vi "Test_WriteCluster_CheckDisk_ValuePresent.vi"(8 "error in (no error)":errorcluster, 11 "TestCase in":refnum<class "TestPersistToDiskTransport.lvclass">) -> (0 "error out":errorcluster, 3 "TestCase out":refnum<class "TestPersistToDiskTransport.lvclass">)   [LabVIEW 2017, in "TestPersistToDiskTransport.lvclass"]
uses:
  TestPersistToDiskTransport.lvclass
  TestPersistToDiskTransport.lvclass/TestPersistToDiskTransport.ctl
  Source/Concrete/PersistToDiskTransport/PersistToDiskTransport.lvclass/PersistToDiskTransport.ctl
  <vilib>/Utility/error.llb/Clear Errors.vi
  Source/Concrete/PersistToDiskTransport/Format Persistent Filename.vi
  Source/Concrete/PersistToDiskTransport/PersistToDiskTransport.lvclass
  C:/Git/composed-transport/Source/ITransport/ITransport.lvclass
  externals/variant-extensions/Source/Format Type String.vi
  Source/ITransport/ITransport.lvclass
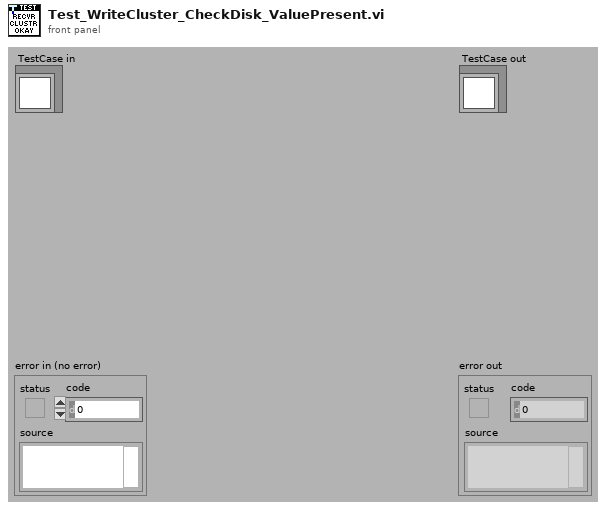
[diagram p1: front panel]
types:
  T1 = typedef "PersistToDiskTransport.lvclass/Recovered Value.ctl" = cluster{"Datum Name":string, "Datum Value":variant, "Last Publication Time":timestamp}
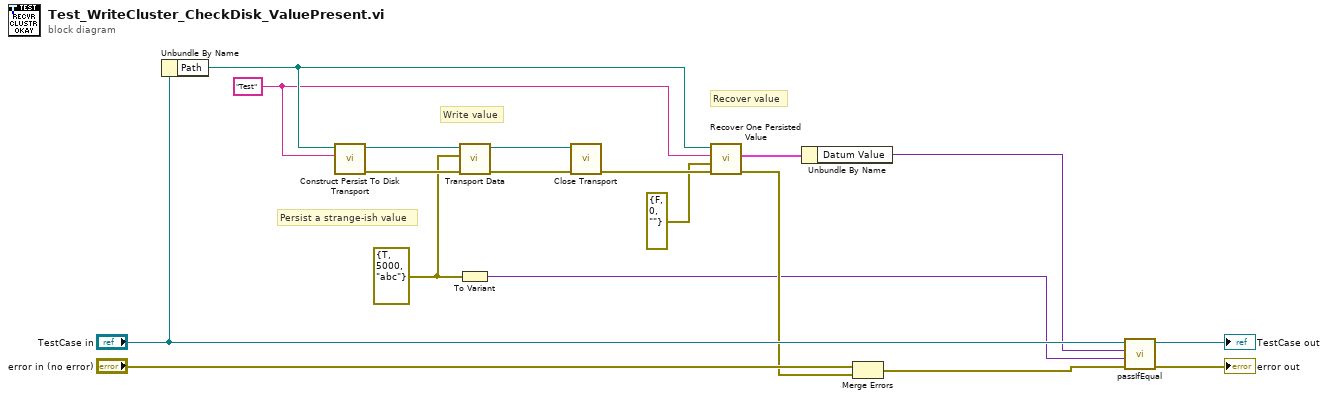
[diagram p0: block diagram]
diagram:
  w8 = "Test" ("Section Name")
  w2 = errorcluster {"status"=TRUE, "code"=5000, "source"="abc"} ("Test Value")
  # "Recover value"
  # "Write value"
  # "Persist a strange-ish value"
  n1 = Unbundle By Name("TestCase in") -> ("Path"=w9:path)
  n2 = call "Construct Persist To Disk Transport.vi"("Datum Name"=w8, "Folder Path"=w9) -> ("error out"=w18:errorcluster, "PersistToDiskTransport"=w12:refnum<class "PersistToDiskTransport.lvclass">)  [unwired: 8 in]
  n3 = call "Transport Data.vi"("error in (no error)"=w18, "Value"=w2, "ITransport in"=w12) -> ("error out"=w10:errorcluster, "ITransport out"=w17:refnum<class "PersistToDiskTransport.lvclass">)  [unwired: 7 in]
  n4 = To Variant(anything=w2) -> (Variant=w1:variant)
  n5 = call-dynamic "Close Transport.vi"("error in (no error)"=w10, "ITransport in"=w17) -> ("error out"=w7:errorcluster)  [unwired: 9 in]
  n6 = call "Recover One Persisted Value.vi"("error in (no error)"=w7, "Data Type"=errorcluster {"status"=FALSE, "code"=0, "source"=""} ("Test Value"), "Datum Name"=w8, "Folder Path"=w9) -> ("error out"=w5:errorcluster, "Recovered Value"=w4:T1)  [unwired: 6 in]
  n7 = Unbundle By Name(w4) -> ("Datum Value"=w3:variant)
  n8 = Merge Errors("error in (no error)", w5) -> (w13:errorcluster)
  n9 = call-dynamic "passIfEqual.vi"("error in (no error)"=w13, "y"=w1, "x"=w3, "TestCase in"="TestCase in") -> ("error out"=→"error out":errorcluster, "TestCase out"=→"TestCase out":refnum<class "TestPersistToDiskTransport.lvclass">)  [unwired: 6 in]
